vi "SplitSubjectToSubstrings.vi"(1 "offsets past match":i32[](array[numeric]), 2 "match offsets":i32[](array[numeric]), 3 "String":string) -> (0 "substrings":string[](array[string]))   [LabVIEW 2021, in "libpcre2-8.lvlib"]
doc: "Splits the subject string into the substrings."
uses:
  libpcre2-8.lvlib
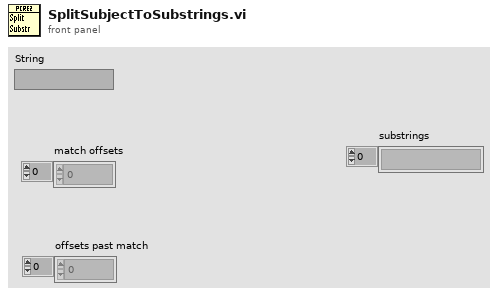
[diagram p1: front panel]
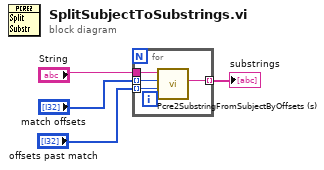
[diagram p0: block diagram]
diagram:
  n1 = for {
    tunnel: "String" -> [w8]
    tunnel: [w5] -> w3 mode=indexing
    tunnel: "match offsets" -> [w7] mode=indexing
    tunnel: "offsets past match" -> [w6] mode=indexing
    n2 = call "Pcre2SubstringFromSubjectByOffsets (s).vi"("OffsetPastMatch"=w6, "MatchOffset"=w7, "Subject"=w8) -> ("Substring"=w5:string)  [unwired: 8 in]
  }
  "substrings" <- w3
